vi "convert_FIFO_data.vi"(0 "Actual Data":i16[](array[numeric])) -> (19 "appended array":dbl[][](array[numeric]))   [LabVIEW 2023]
uses:
  I32Dim_to_umDim.vi
  User_Vi/Settings.vi
panel:
  out "size(s)":i32
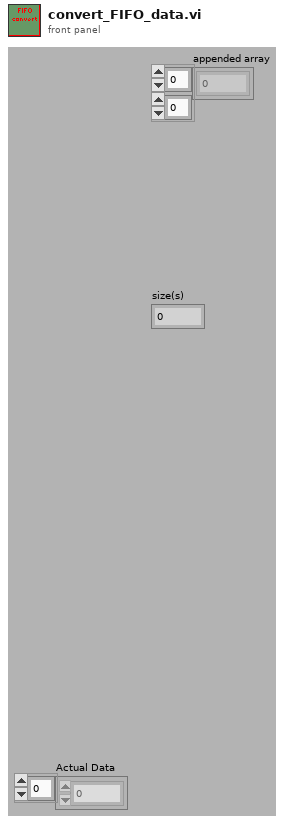
[diagram p1: front panel]
types:
  T1 = typedef "Current Amplifier Settings.ctl" = dbl
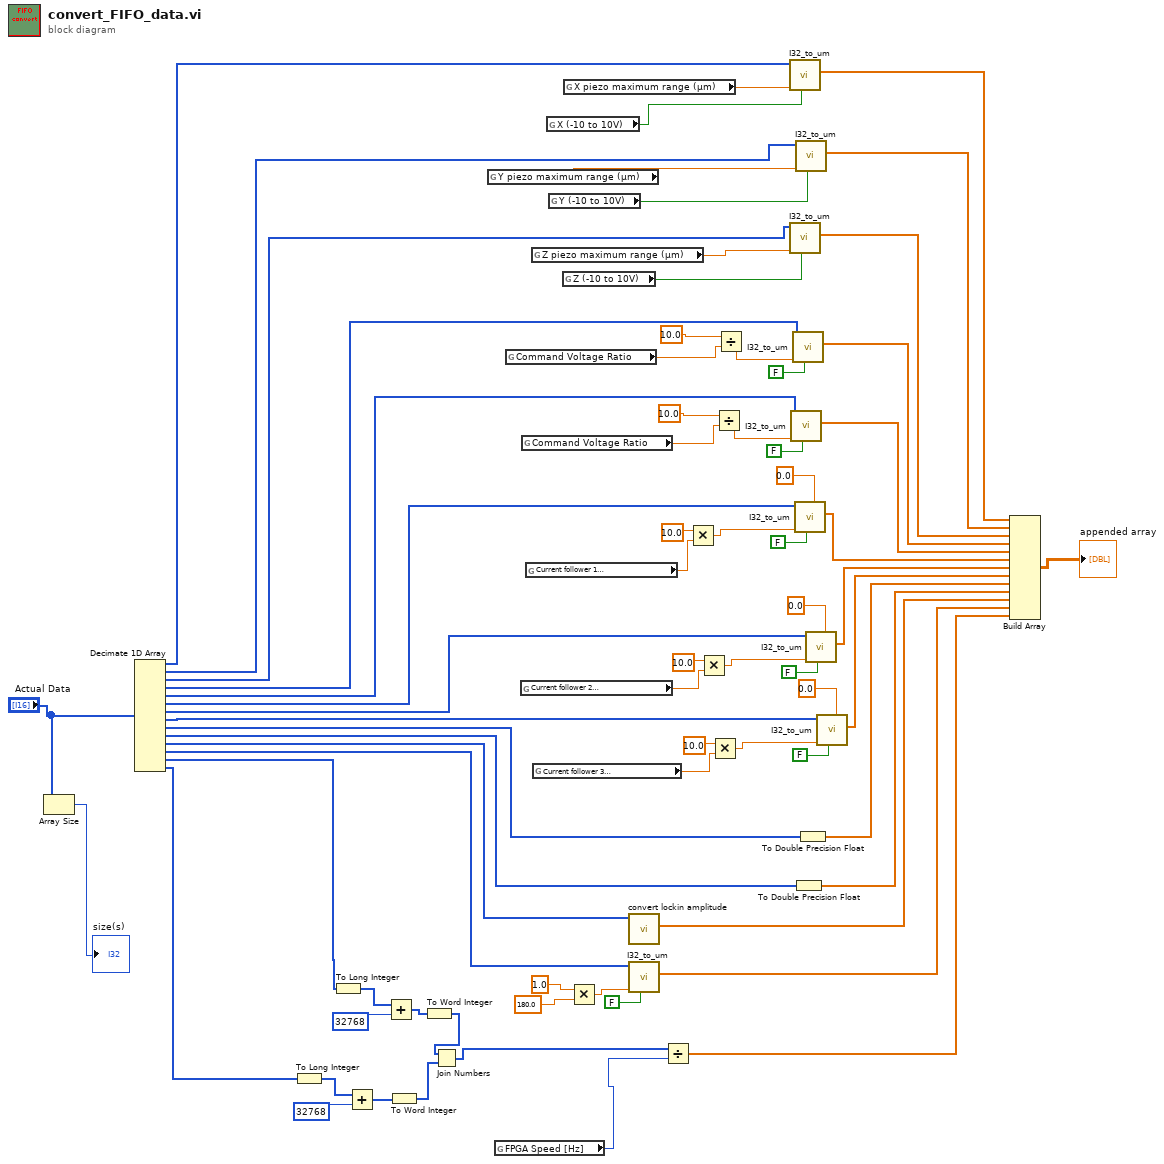
[diagram p0: block diagram]
diagram:
  n1 = Array Size(array="Actual Data") -> (size(s)=→"size(s)":i32)
  n2 = Decimate 1D Array("Actual Data") -> (w60:i16[], w59:i16[], w58:i16[], w56:i16[], w52:i16[], w51:i16[], w46:i16[], w41:i16[], w40:i16[], w39:i16[], w38:i16[], w37:i16[], w21:i16[], w16:i16[])
  n3 = To Long Integer(number=w16) -> (32bit integer=w17:i32[])
  n4 = To Long Integer(number=w21) -> (32bit integer=w20:i32[])
  n5 = Add(x=w17, y=32768 ("Max Value [um]")) -> (x+y=w13:i32[])
  n6 = Add(x=w20, y=32768 ("Max Value [um]")) -> (x+y=w14:i32[])
  n7 = To Word Integer(number=w13) -> (16bit integer=w12:i16[])
  n8 = To Word Integer(number=w14) -> (16bit integer=w11:i16[])
  n9 = Join Numbers(hi=w11, lo=w12) -> ((hi.lo)=w15:u32[])
  n10 = global read "Settings.vi" "Y piezo maximum range (µm)"() -> (w57:dbl)
  n11 = global read "Settings.vi" "FPGA Speed [Hz]"() -> (w9:i64)
  n12 = global read "Settings.vi" "Command Voltage Ratio"() -> (w5:dbl)
  n13 = global read "Settings.vi" "Current follower 2 \n(AI-4)"() -> (w49:T1)
  n14 = global read "Settings.vi" "Command Voltage Ratio"() -> (w4:dbl)
  n15 = global read "Settings.vi" "Current follower 1\n (AI-3)"() -> (w62:T1)
  n16 = global read "Settings.vi" "Z piezo maximum range (µm)"() -> (w73:dbl)
  n17 = global read "Settings.vi" "Current follower 3\n(AI-6)"() -> (w43:T1)
  n18 = global read "Settings.vi" "X (-10 to 10V)"() -> (w8:bool)
  n19 = global read "Settings.vi" "Y (-10 to 10V)"() -> (w7:bool)
  n20 = global read "Settings.vi" "Z (-10 to 10V)"() -> (w6:bool)
  n21 = global read "Settings.vi" "X piezo maximum range (µm)"() -> (w68:dbl)
  n22 = Multiply(x=1.0, y=180.0) -> (x*y=w71:dbl)
  n23 = call "convert lockin amplitude.vi"("Input"=w38) -> ("x*y"=w26:dbl[])  [unwired: 10 in]
  n24 = call-poly "I32_to_um.vi"("-10 to 10V range?"=FALSE, "Max Value [um]"=w71, "Input"=w37) -> ("x*y"=w25:dbl[])  [unwired: 8 in]
  n25 = Divide(x=w15, y=w9) -> (x/y=w22:dbl[])
  n26 = Multiply(x=10.0 ("Max Value [um]"), y=w62) -> (x*y=w61:T1)
  n27 = Multiply(x=10.0 ("Max Value [um]"), y=w49) -> (x*y=w50:T1)
  n28 = Multiply(x=10.0 ("Max Value [um]"), y=w43) -> (x*y=w42:T1)
  n29 = Divide(x=10.0 ("Max Value [um]"), y=w4) -> (x/y=w55:dbl)
  n30 = Divide(x=10.0 ("Max Value [um]"), y=w5) -> (x/y=w64:dbl)
  n31 = call-poly "I32_to_um.vi"("-10 to 10V range?"=w8, "Max Value [um]"=w68, "Input"=w60) -> ("x*y"=w36:dbl[])  [unwired: 8 in]
  n32 = call-poly "I32_to_um.vi"("-10 to 10V range?"=w6, "Max Value [um]"=w73, "Input"=w58) -> ("x*y"=w34:dbl[])  [unwired: 8 in]
  n33 = call-poly "I32_to_um.vi"("-10 to 10V range?"=FALSE, "Max Value [um]"=w55, "Input"=w52) -> ("x*y"=w32:dbl[])  [unwired: 8 in]
  n34 = call-poly "I32_to_um.vi"("-10 to 10V range?"=FALSE, "Max Value [um]"=w64, "Input"=w56) -> ("x*y"=w33:dbl[])  [unwired: 8 in]
  n35 = To Double Precision Float(number=w39) -> (double precision float=w27:dbl[])
  n36 = call-poly "I32_to_um.vi"("Offset"=0.0, "-10 to 10V range?"=FALSE, "Max Value [um]"=w61, "Input"=w51) -> ("x*y"=w31:dbl[])  [unwired: 7 in]
  n37 = call-poly "I32_to_um.vi"("-10 to 10V range?"=w7, "Max Value [um]"=w57, "Input"=w59) -> ("x*y"=w35:dbl[])  [unwired: 8 in]
  n38 = To Double Precision Float(number=w40) -> (double precision float=w28:dbl[])
  n39 = call-poly "I32_to_um.vi"("Offset"=0.0, "-10 to 10V range?"=FALSE, "Max Value [um]"=w50, "Input"=w46) -> ("x*y"=w30:dbl[])  [unwired: 7 in]
  n40 = call-poly "I32_to_um.vi"("Offset"=0.0, "-10 to 10V range?"=FALSE, "Max Value [um]"=w42, "Input"=w41) -> ("x*y"=w29:dbl[])  [unwired: 7 in]
  n41 = Build Array(w36, w35, w34, w33, w32, w31, w30, w29, w28, w27, w26, w25, w22) -> (→"appended array":dbl[][])
